vi "TestClearAll.vi"   [LabVIEW 2017]
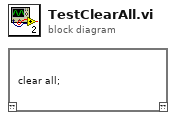
[diagram p0: block diagram]
diagram:
  n1 = script code="clear all;"() -> ()  [unwired: 1 in, 1 out]
